vi "Mettler Toledo Test.vi"() -> ()   [LabVIEW 2018, in "Mettler Toledo.lvlib"]
uses:
  Mettler Toledo.lvlib
  Controls/Settings Cluster.ctl
panel:
  out "error out":errorcluster
  out "Mettler Settings out":T1
  in  "Mettler Settings in":T1
  in  "stop":bool
  out "Connection Error":bool
  out "mass (g)":dbl
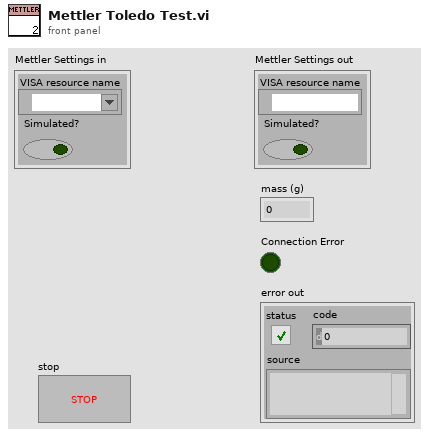
[diagram p1: front panel]
types:
  T1 = typedef "Mettler Toledo.lvlib/Settings Cluster.ctl" = cluster{"VISA resource name":refnum<visa-resource-name>, "Simulated?":bool}
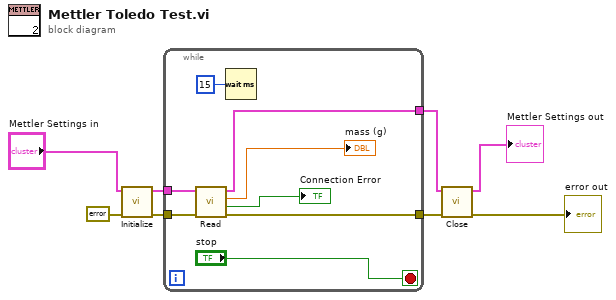
[diagram p0: block diagram]
diagram:
  n1 = call "Initialize.vi"("error in (no error)"=errorcluster {"status"=FALSE, "code"=0, "source"=""}, "Mettler Settings in"="Mettler Settings in") -> ("error out"=w7:errorcluster, "Mettler Settings out"=w8:T1)  [unwired: 7 in, 1 out]
  n2 = while {
    tunnel: w8 -> [w16]
    tunnel: w7 -> [w15]
    tunnel: [w14] -> w6
    tunnel: [w13] -> w5
    stop <- "stop" stop-if-true
    n3 = call "Read.vi"("error in (no error)"=w15, "Mettler Settings in"=w16) -> ("error out"=w13:errorcluster, "Connection Error"=→"Connection Error":bool, "mass (g)"=→"mass (g)":dbl, "Mettler Settings out"=w14:T1)  [unwired: 6 in]
    n4 = Wait (ms)(milliseconds to wait=u32 15) -> ()  [unwired: 1 out]
  }
  n5 = call "Close.vi"("error in (no error)"=w5, "Mettler Settings in"=w6) -> ("error out"=→"error out":errorcluster, "Mettler Settings out"=→"Mettler Settings out":T1)  [unwired: 8 in]
